vi "Set Pulse Mode.vi"(8 "error in (no error)":errorcluster, 10 "pulse mode (CW)":T1) -> (0 "error out":errorcluster, 2 "return value":u32)   [LabVIEW 2009, in "HighFinesse WS5.lvlib"]
doc: "Sets the pulse mode for the wavelength meter."
uses:
  HighFinesse WS5.lvlib
  Control typedefs.llb/Pulse Mode.ctl
  WINDOWS/system32/wlmData.dll
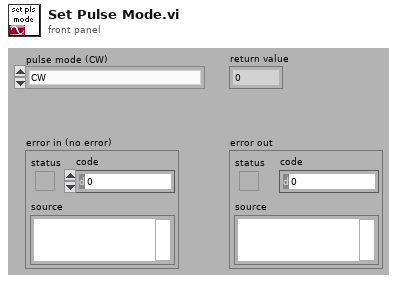
[diagram p1: front panel]
types:
  T1 = typedef "HighFinesse WS5.lvlib/Pulse Mode.ctl" = enum16{"CW", "pulsed (standard)", "single pulsed (MLC)", "single pulsed (int trigger)", "single pulsed (ext trigger)", "double pulsed (TTL-triggered)", "double pulsed (optically triggered)"}
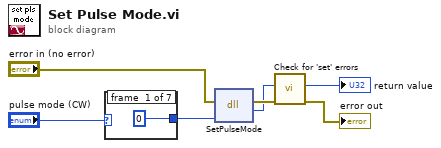
[diagram p0: block diagram]
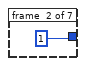
[diagram p2: hidden frame]
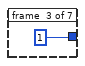
[diagram p3: hidden frame]
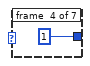
[diagram p4: hidden frame]
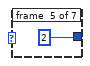
[diagram p5: hidden frame]
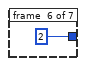
[diagram p6: hidden frame]
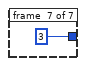
[diagram p7: hidden frame]
diagram:
  n1 = case shown="\"CW\", Default" "pulse mode (CW)" {
    tunnel: [u8 0 ("Res1") u8 1 ("Res1") u8 1 ("Res1") u8 1 ("Res1") u8 2 ("Res1") u8 2 ("Res1") u8 3 ("Res1")] -> w1
    frame #0 {
    }
    frame #1 {
    }
    frame #2 {
    }
    frame #3 {
    }
    frame #4 {
    }
    frame #5 {
    }
    frame #6 {
    }
  }
  n2 = dll-call lib="C:/WINDOWS/system32/wlmData.dll" fn="SetPulseMode"(error in="error in (no error)", "PM"=w1) -> (error out=w5:errorcluster, "return type"=w3:u32)  [unwired: 3 in, 1 out]
  n3 = call "Check for 'set' errors.vi"("error in (no error)"=w5, "return value"=w3) -> ("error out"=→"error out":errorcluster, "return value out"=→"return value":i32)  [unwired: 8 out]
